vi "Read.vi"(8 "error out":errorcluster caption="error in", 10 "Read":T1={"Index"="``", "Sub-Index"="\u0000", "Data-Size (in Byte)"=1, FALSE} {"Data-Size (in Byte)" min=1 max=4 step=1 format="%x"}, 11 "ComPort In":refnum<visa-resource-name>) -> (0 "error out 2":errorcluster caption="error out", 2 "Answer":i32, 3 "ComPort Out":refnum<visa-resource-name>)   [LabVIEW 2021]
panel:
  out "read buffer":string
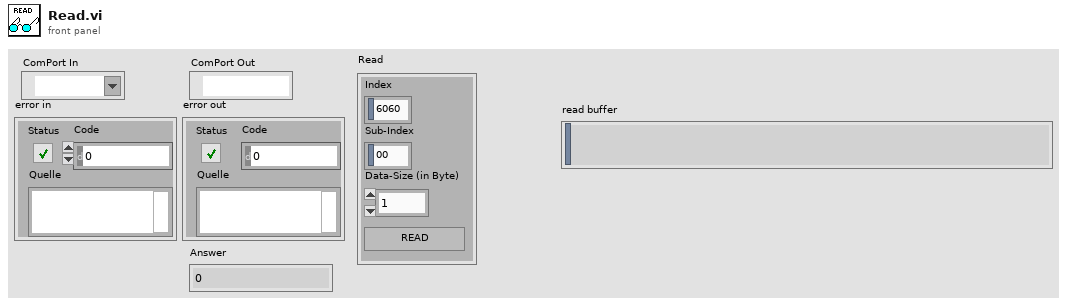
[diagram p1: front panel]
types:
  T1 = cluster{"Index":string, "Sub-Index":string, "Data-Size (in Byte)":u8, bool}
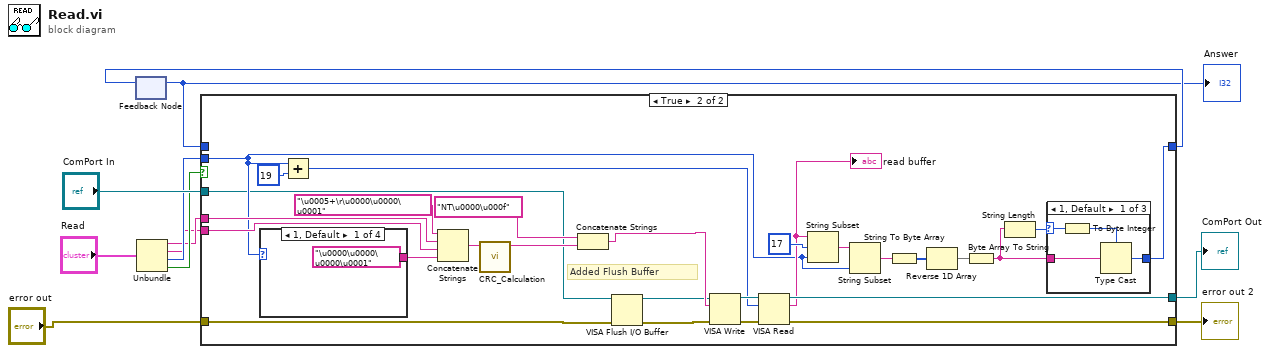
[diagram p0: block diagram]
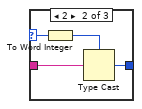
[diagram p3: hidden frame]
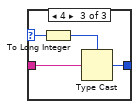
[diagram p4: hidden frame]
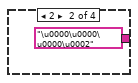
[diagram p5: hidden frame]
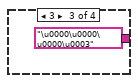
[diagram p6: hidden frame]
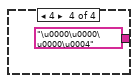
[diagram p7: hidden frame]
diagram:
  n1 = feedback #1() -> (w9:i32)  [unwired: 1 in]
  "Answer" <- w9
  n2 = Unbundle("Read") -> ("Index"=w3:string, "Sub-Index"=w2:string, "Data-Size (in Byte)"=w4:u8, w5:bool)
  n3 = case shown="True" w5 {
    tunnel: "ComPort In" -> [w13 w19]
    tunnel: "error out" -> [w14 w17]
    tunnel: [w14 w37] -> w11
    tunnel: w4 -> [_ w20]
    tunnel: w3 -> [_ w36]
    tunnel: w2 -> [_ w35]
    tunnel: [w13 w31] -> w7
    tunnel: [w12 w22] -> w10
    tunnel: w9 -> [w12 _]
    frame False {
    }
    frame True {
      # "Added Flush Buffer"
      n4 = case shown="1, Default" w20 {
        tunnel: ["\u0000\u0000\u0000\u0001" ("Hexadecimal Input String 4") "\u0000\u0000\u0000\u0002" ("Hexadecimal Input String 4") "\u0000\u0000\u0000\u0003" ("Hexadecimal Input String 4") "\u0000\u0000\u0000\u0004" ("Hexadecimal Input String 4")] -> w30
        frame 1, Default {
        }
        frame 2 {
        }
        frame 3 {
        }
        frame 4 {
        }
      }
      n5 = Add(x=w20, y=u32 19 ("byte count")) -> (x+y=w32:u32)
      n6 = Concatenate Strings("\u0005+\r\u0000\u0000\u0001" ("Hexadecimal Input String 4"), w36, w35, w30) -> (w39:string)
      n7 = call "CRC_Calculation.vi"("CMD"=w39) -> ("CMD + CRC"=w38:string)  [unwired: 10 in]
      n8 = Concatenate Strings("NT\u0000\u000f" ("Hexadecimal Input String 4"), w38) -> (w18:string)
      n9 = VISA Flush I/O Buffer(VISA resource name=w19, error in (no error)=w17) -> (VISA resource name out=w15:refnum<visa-resource-name>, error out=w16:errorcluster)  [unwired: 1 in]
      n10 = VISA Write(VISA resource name=w15, write buffer=w18, error in (no error)=w16) -> (VISA resource name out=w41:refnum<visa-resource-name>, error out=w42:errorcluster)  [unwired: 1 out]
      n11 = VISA Read(VISA resource name=w41, byte count=w32, error in (no error)=w42) -> (VISA resource name out=w31:refnum<visa-resource-name>, read buffer=w21:string, error out=w37:errorcluster)  [unwired: 1 out]
      "read buffer" <- w21
      n12 = String Subset(string=w21, offset (0)=u8 17 ("x"), length (rest)=w20) -> (substring=w24:string)
      n13 = String Subset(string=w24, length (rest)=w20) -> (substring=w27:string)  [unwired: 1 in]
      n14 = String To Byte Array(string=w27) -> (unsigned byte array=w26:u8[])
      n15 = Reverse 1D Array(array=w26) -> (reversed array=w25:u8[])
      n16 = Byte Array To String(unsigned byte array=w25) -> (string=w29:string)
      n17 = String Length(string=w29) -> (length=w28:i32)
      n18 = case shown="1, Default" w28 {
        selector: w28 -> [w46 w50 w54]
        tunnel: w29 -> [w43 w48 w53]
        tunnel: [w44 w47 w52] -> w22
        frame 1, Default {
          n19 = To Byte Integer(number=w46) -> (8bit integer=w45:i8)
          n20 = Type Cast(type=w45, x=w43) -> (*(type *) &x=w44:i8)
        }
        frame 2 {
          n21 = To Word Integer(number=w50) -> (16bit integer=w49:i16)
          n22 = Type Cast(type=w49, x=w48) -> (*(type *) &x=w47:i16)
        }
        frame 4 {
          n23 = To Long Integer(number=w54) -> (32bit integer=w51:i32)
          n24 = Type Cast(type=w51, x=w53) -> (*(type *) &x=w52:i32)
        }
      }
    }
  }
  "error out 2" <- w11
  "ComPort Out" <- w7
  n25 = feedback-in #1(w10) -> ()
